vi "init_http_client.vi"(6 "timeout (ms)":i32=10000, 8 "error in (no error)":errorcluster, 9 "password":string, 10 "username":string, 11 "IP address":string) -> (0 "error out":errorcluster, 2 "token cluster":T2, 3 "client handle out":T1)   [LabVIEW 2018]
uses:
  <vilib>/httpClient/ClientHandle.ctl
  <vilib>/httpClient/POSTBuffer.vi
  <vilib>/httpClient/LabVIEWHTTPClient.lvlib
panel:
  out "headers":string
  out "code":string
  out "msg":string
  out "reponse":string
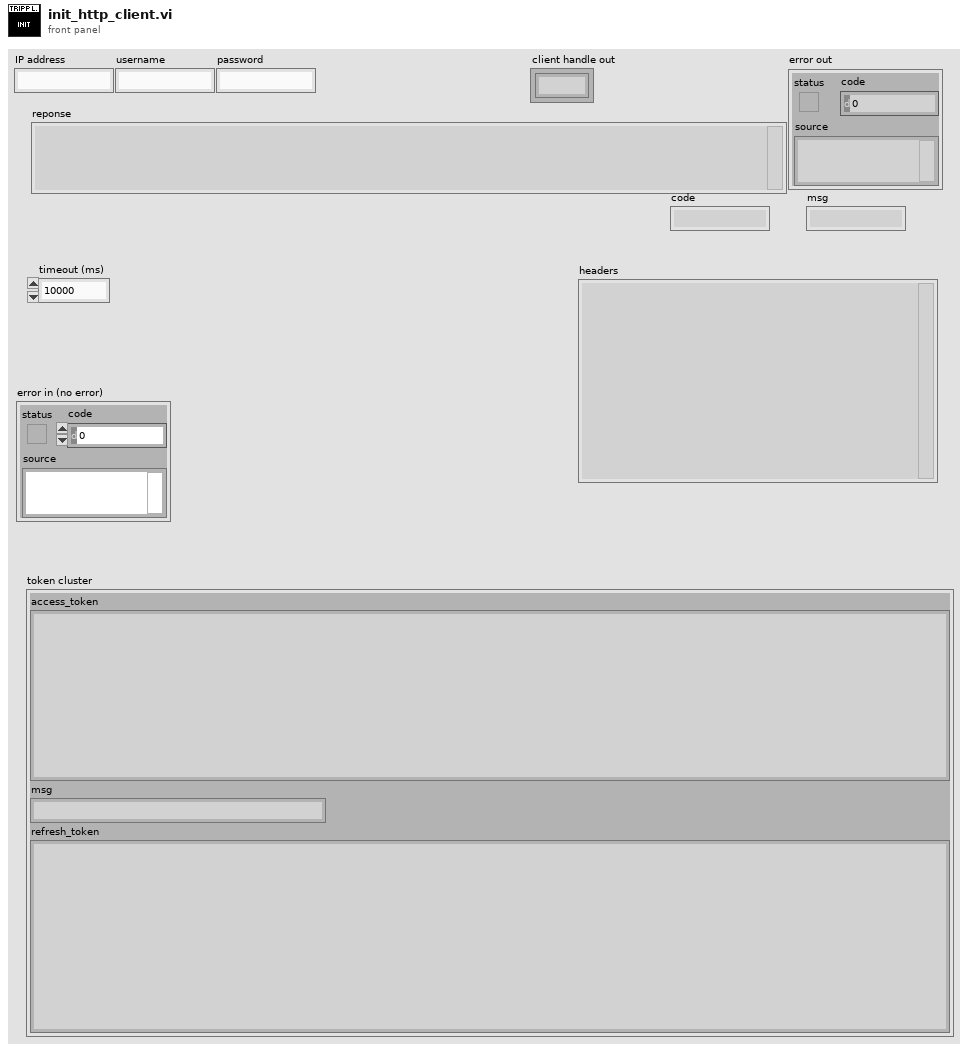
[diagram p1: front panel]
types:
  T1 = typedef "LabVIEWHTTPClient.lvlib/ClientHandle.ctl" = refnum<k1>
  T2 = cluster{"access_token":string, "msg":string, "refresh_token":string}
  T3 = cluster{"username":string, "password":string, "grant_type":string}
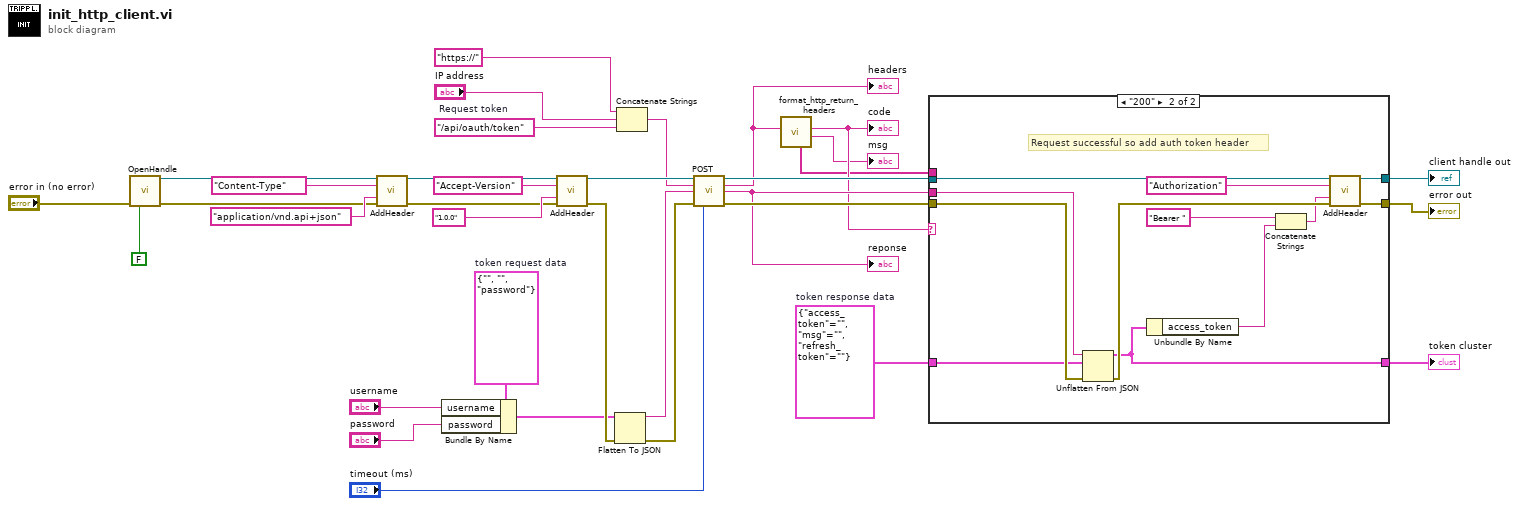
[diagram p0: block diagram]
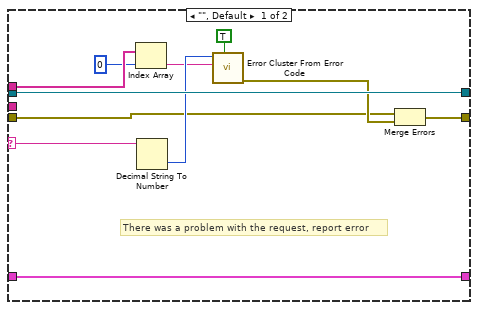
[diagram p2: hidden frame]
diagram:
  w5 = T2 {"access_token"="", "msg"="", "refresh_token"=""}  # token response data
  w17 = "/api/oauth/token"  # Request token
  w10 = T3 {"username"="", "password"="", "grant_type"="password"}  # token request data
  n1 = call <vilib>:"OpenHandle.vi"("error in (no error)"="error in (no error)", "verify server(true)"=FALSE) -> ("client handle out"=w30:T1, "error out"=w29:errorcluster)  [unwired: 12 in]
  n2 = call <vilib>:"AddHeader.vi"("client handle"=w30, "header"="Content-Type", "value"="application/vnd.api+json", "error in (no error)"=w29) -> ("client handle out"=w28:T1, "error out"=w27:errorcluster)  [unwired: 10 in]
  n3 = Bundle By Name(cluster=w10, "username"="username", "password"="password") -> (w7:T3)
  n4 = call <vilib>:"AddHeader.vi"("client handle"=w28, "header"="Accept-Version" ("value"), "value"="1.0.0", "error in (no error)"=w27) -> ("client handle out"=w26:T1, "error out"=w24:errorcluster)  [unwired: 10 in]
  n5 = Flatten To JSON(anything=w7, error in (no error)=w24) -> (JSON string=w19:string, 11:w23:errorcluster)  [unwired: 1 in]
  n6 = Concatenate Strings("https://", "IP address", w17) -> (w25:string)
  n7 = call-poly <vilib>:"POST.vi"("client handle"=w26, "url"=w25, "buffer"=w19, "error in (no error)"=w23, "timeout (10000)"="timeout (ms)") -> ("client handle out"=w18:T1, "headers"=w11:string, "body"=w21:string, "error out"=w22:errorcluster)  [unwired: 7 in]
  "reponse" <- w21
  "headers" <- w11
  n8 = call "format_http_return_headers.vi"("headers in"=w11) -> ("msg"=→"msg":string, "status code"=w6:string, "headers array"=w2:string[])  [unwired: 8 in]
  "code" <- w6
  n9 = case shown="\"200\"" w6 {
    selector: w6 -> [w41 _]
    tunnel: w22 -> [w36 w57]
    tunnel: w21 -> [_ w56]
    tunnel: w18 -> [w45 w54]
    tunnel: [w35 w49] -> w13
    tunnel: [w45 w48] -> w12
    tunnel: w5 -> [w44 w47]
    tunnel: [w44 w46] -> w4
    tunnel: w2 -> [w40 _]
    frame "", Default {
      # "There was a problem with the request, report error"
      n10 = Index Array(array=w40, index=0) -> (element=w38:string)
      n11 = Decimal String To Number(string=w41) -> (number=w42:i32)  [unwired: 2 in, 1 out]
      n12 = call <vilib>:"Error Cluster From Error Code.vi"("show call chain? (False)"=TRUE, "error message (\"\")"=w38, "error code (0)"=w42) -> ("error out"=w37:errorcluster)  [unwired: 6 in]
      n13 = Merge Errors(w36, w37) -> (w35:errorcluster)
    }
    frame "200" {
      # "Request successful so add auth token header"
      n14 = Unflatten From JSON(JSON string=w56, type and defaults=w47, error in (no error)=w57) -> (value=w46:T2, error out=w55:errorcluster)  [unwired: 4 in]
      n15 = Unbundle By Name(w46) -> ("access_token"=w51:string)
      n16 = Concatenate Strings("Bearer " ("value"), w51) -> (w50:string)
      n17 = call <vilib>:"AddHeader.vi"("client handle"=w54, "header"="Authorization" ("value"), "value"=w50, "error in (no error)"=w55) -> ("client handle out"=w48:T1, "error out"=w49:errorcluster)  [unwired: 10 in]
    }
  }
  "error out" <- w13
  "client handle out" <- w12
  "token cluster" <- w4
